vi "Column Letter To Number.vi"(8 "error in":errorcluster, 11 "Letter":string) -> (0 "error out":errorcluster, 3 "Number":i32)   [LabVIEW 2020, in "Open Xml.lvlib"]
uses:
  Open Xml.lvlib
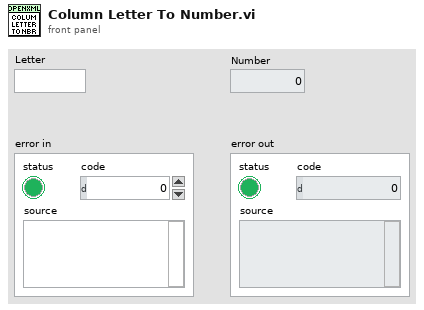
[diagram p1: front panel]
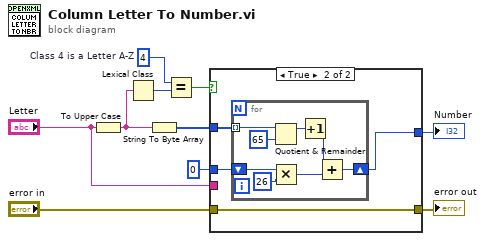
[diagram p0: block diagram]
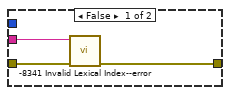
[diagram p2: hidden frame]
diagram:
  w9 = i16 4  # Class 4 is a Letter A-Z
  n1 = To Upper Case(1:"Letter") -> (0:w4:string)
  n2 = Lexical Class(1:w4) -> (0:w10:i16)
  n3 = String To Byte Array(string=w4) -> (unsigned byte array=w3:u8[])
  n4 = Equal?(x=w9, y=w10) -> (x = y?=w5:bool)
  n5 = case shown="True" w5 {
    tunnel: "error in" -> [w13 w16]
    tunnel: [w12 w16] -> w7
    tunnel: "Letter" -> [w11 _]
    tunnel: w3 -> [_ w17]
    tunnel: 0 ("y") -> [_ w15]
    tunnel: [_ w14] -> w1
    frame False {
      n6 = call "-8341 Invalid Lexical Index--error.vi"("error in"=w13, "Lexical Index"=w11) -> ("error out"=w12:errorcluster)  [unwired: 9 in]
    }
    frame True {
      n7 = for {
        tunnel: w17 -> [w24] mode=indexing
        shift-right: [w18] -> w14
        shift-left: w15 -> [w22]
        n8 = Quotient & Remainder(x=w24, y=u8 65) -> (x-y*floor(x/y)=w23:u8)  [unwired: 1 out]
        n9 = Multiply(x=w22, y=26) -> (x*y=w21:i32)
        n10 = Increment(x=w23) -> (x+1=w20:u8)
        n11 = Add(x=w20, y=w21) -> (x+y=w18:i32)
      }
    }
  }
  "error out" <- w7
  "Number" <- w1
